vi "MU Activate Mt Sync Config.vi"(8 "error in (no error)":errorcluster, 11 "MUhandle":u64) -> (0 "error out":errorcluster, 3 "function return":u32)   [LabVIEW 2017, in "MU_3SL_interface.lvlib"]
uses:
  MU_3SL_interface.lvlib
  lib/MU_3SL_interface.dll
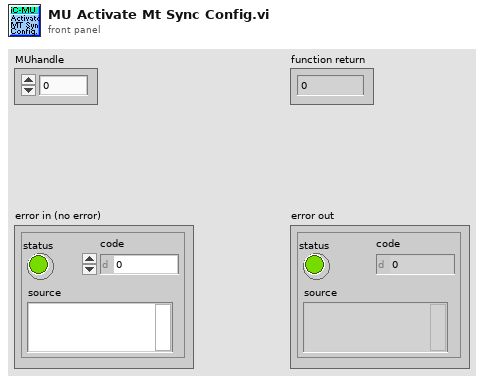
[diagram p1: front panel]
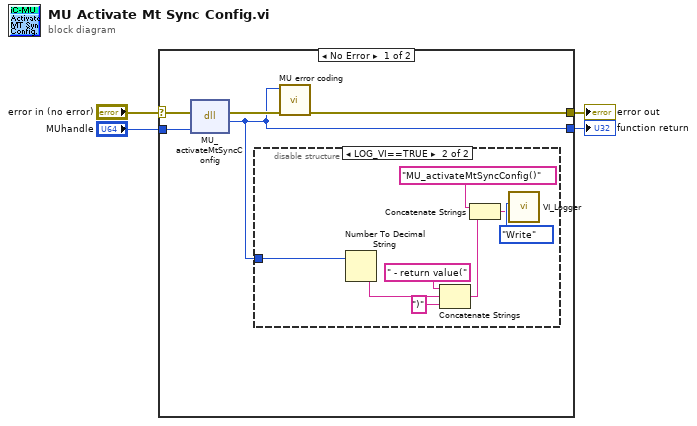
[diagram p0: block diagram]
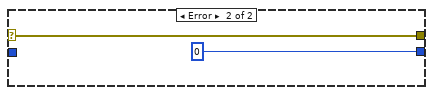
[diagram p3: hidden frame]
diagram:
  n1 = case shown="No Error" "error in (no error)" {
    selector: "error in (no error)" -> [w7 w19]
    tunnel: [w5 u32 0] -> w4
    tunnel: [w8 w19] -> w3
    tunnel: "MUhandle" -> [w6 _]
    frame No Error {
      n2 = dll-call lib="C:/Users/bes/AppData/Roaming/work/mu_9so/icsubmodules/soft_mu_3sl_master/lv_interface/lib/MU_3SL_interface**.*" fn="MU_activateMtSyncConfig"(error in=w7, "handle"=w6) -> (error out=w9:errorcluster, "return type"=w5:u32)  [unwired: 3 in, 1 out]
      n3 = disable-structure shown="LOG_VI==TRUE" {
        disable-tunnel: w5 -> [_ w11]
        frame condition #0 {
        }
        frame condition #1 (active) {
          n4 = Number To Decimal String(number=w11) -> (decimal integer string=w10:string)  [unwired: 1 in]
          n5 = Concatenate Strings(" - return value(" ("string"), w10, ")" ("string")) -> (w15:string)
          n6 = Concatenate Strings("MU_activateMtSyncConfig()" ("Info in"), w15) -> (w14:string)
          n7 = call "VI_Logger.vi"("Action (Read)"=enum16{"Write", "Read"}."Write", "Info in"=w14) -> ()  [unwired: 8 in, 2 out]
        }
      }
      n8 = call "MU error coding.vi"("error in (no error)"=w9, "function return in"=w5) -> ("error out"=w8:errorcluster)  [unwired: 9 in]
    }
    frame Error {
    }
  }
  "function return" <- w4
  "error out" <- w3
